vi "Diagram Disable Structure.vi"() -> ()   [LabVIEW 2023]
doc: "Diagram Disable Structures are used to \"comment out\" code in the block diagram. Any code that is within the \"Disabled\" subdiagram of a given Diagram Disable Structure is not compiled or checked for errors."
panel:
  in  "Y":i32=2
  in  "X":i32=1
  out "Result":i32
  # "Overview: Demonstrates the use of a Diagram Disable Structure to comment out a section of code on the block diagram.\nInstructions:\nRun the VI. Even though there is a broken wire in this code, it still executes. See the block diagram for more information."
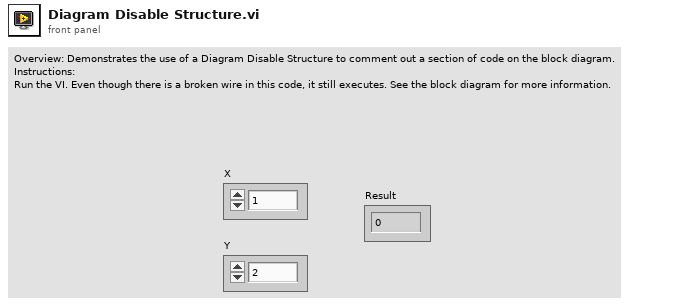
[diagram p1: front panel]
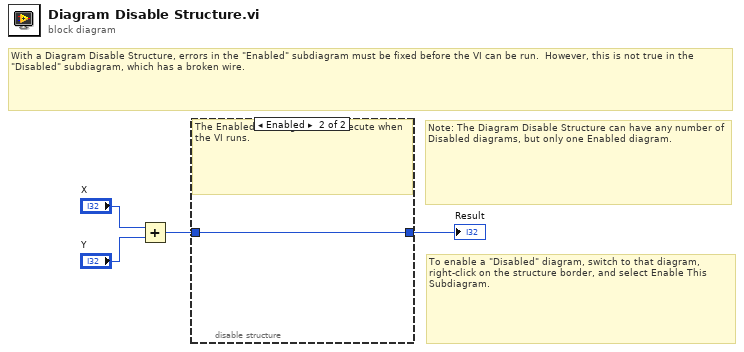
[diagram p0: block diagram]
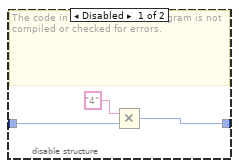
[diagram p2: hidden frame]
diagram:
  # "To enable a \"Disabled\" diagram, switch to that diagram, right-click on the structure border, and select Enable This Subdiagram."
  # "With a Diagram Disable Structure, errors in the \"Enabled\" subdiagram must be fixed before the VI can be run.  However, this is not true in the \"Disabled\" subdiagram, which has a broken wire."
  # "Note: The Diagram Disable Structure can have any number of Disabled diagrams, but only one Enabled diagram."
  n1 = Add(x="X", y="Y") -> (x+y=w2:i32)
  n2 = disable-structure "Diagram Disable Structure" shown="Enabled" {
    disable-tunnel: w2 -> [w7 w8]
    disable-tunnel: [w6 w8] -> w1
    frame Disabled {
      # "The code in the Disabled subdiagram is not compiled or checked for errors."
      n3 = Multiply(x="4" ("Z"), y=w7) -> (x*y=w6:i32)
    }
    frame Enabled {
      # "The Enabled subdiagram will execute when the VI runs."
    }
  }
  "Result" <- w1
